vi "AjustTime.vi"(8 "error in (no error)":errorcluster, 10 "Pomiar in":refnum<k34>, 11 "Test in":refnum<k34>) -> (0 "error out":errorcluster, 2 "Pomiar Out":refnum<k34>, 3 "Test Out":refnum<k34>, 4 "First Pomiar":i64, 5 "FirstTest":i64, 7 "End":i64)   [LabVIEW 2019]
uses:
  App/Global_Freq.vi
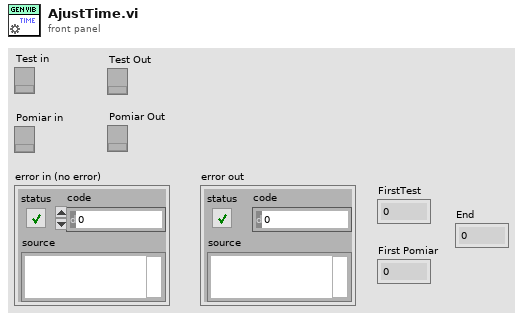
[diagram p1: front panel]
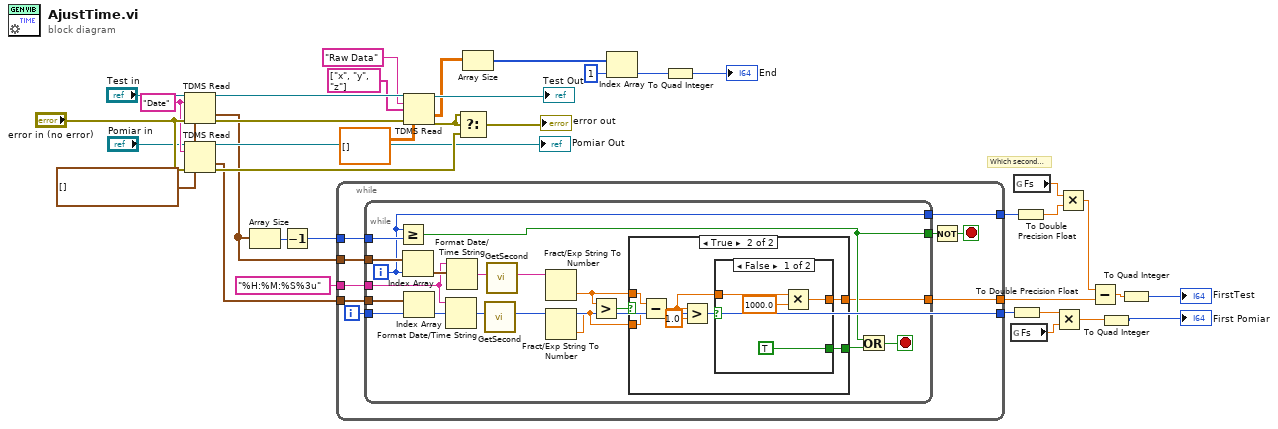
[diagram p0: block diagram]
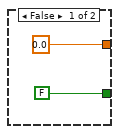
[diagram p2: hidden frame]
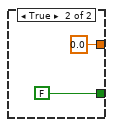
[diagram p3: hidden frame]
diagram:
  w30 = timestamp[] [] ("appended array")
  w34 = "Date" ("group name in")
  # "Which second Test"
  n1 = TDMS Read(0:"Test in", 5:w34, 11:"error in (no error)", 12:w30) -> (4:w29:refnum<k34>, 10:w17:timestamp[], 15:w28:errorcluster)  [unwired: 4 in, 3 out]
  n2 = TDMS Read(0:"Pomiar in", 5:w34, 11:"error in (no error)", 12:w30) -> (4:→"Pomiar Out":refnum<k34>, 10:w19:timestamp[], 15:w35:errorcluster)  [unwired: 4 in, 3 out]
  n3 = Array Size(array=w17) -> (size(s)=w18:i32)
  n4 = Decrement(x=w18) -> (x-1=w16:i32)
  n5 = while {
    tunnel: w19 -> [w46]
    tunnel: w17 -> [w45]
    tunnel: w16 -> [w44]
    tunnel: [w41] -> w15
    tunnel: [w40] -> w12
    tunnel: [w39] -> w8
    tunnel: "%H:%M:%S%3u" ("time format string (%c)") -> [w38]
    i -> [w40]
    stop <- w42 stop-if-true
    n6 = while {
      tunnel: w45 -> [w60]
      tunnel: w46 -> [w59]
      tunnel: w44 -> [w58]
      tunnel: [w55] -> w43
      tunnel: w40 -> [w54]
      tunnel: [w53] -> w41
      tunnel: [w52] -> w39
      tunnel: w38 -> [w47]
      i -> [w53]
      stop <- w56 stop-if-true
      n7 = Greater Or Equal?(x=w53, y=w58) -> (x >= y?=w55:bool)
      n8 = Index Array(array=w60, index=w53) -> (element=w62:timestamp)
      n9 = Index Array(array=w59, index=w54) -> (element=w61:timestamp)
      n10 = Format Date/Time String(time format string (%c)=w47, seconds (now)=w61) -> (date/time string=w49:string)  [unwired: 1 in]
      n11 = Format Date/Time String(time format string (%c)=w47, seconds (now)=w62) -> (date/time string=w51:string)  [unwired: 1 in]
      n12 = call "GetSecond.vi"("String in"=w49) -> ("String out"=w48:string)  [unwired: 10 in]
      n13 = call "GetSecond.vi"("String in"=w51) -> ("String out"=w50:string)  [unwired: 10 in]
      n14 = Fract/Exp String To Number(string=w50) -> (number=w65:dbl)  [unwired: 3 in, 1 out]
      n15 = Fract/Exp String To Number(string=w48) -> (number=w64:dbl)  [unwired: 3 in, 1 out]
      n16 = Greater?(x=w65, y=w64) -> (0:w63:bool)
      n17 = case shown="True" w63 {
        tunnel: w65 -> [_ w71]
        tunnel: w64 -> [_ w70]
        tunnel: [FALSE w69] -> w57
        tunnel: [0.0 w68] -> w52
        frame False {
        }
        frame True {
          n18 = Subtract(x=w71, y=w70) -> (x-y=w72:dbl)
          n19 = Greater?(x=w72, y=1.0) -> (0:w73:bool)
          n20 = case shown="False" w73 {
            tunnel: [TRUE FALSE] -> w69
            tunnel: w72 -> [w77 _]
            tunnel: [w75 0.0] -> w68
            frame False {
              n21 = Multiply(x=w77, y=1000.0) -> (x*y=w75:dbl)
            }
            frame True {
            }
          }
        }
      }
      n22 = Or(x=w55, y=w57) -> (x .or. y?=w56:bool)
    }
    n23 = Not(x=w43) -> (.not. x?=w42:bool)
  }
  n24 = TDMS Read(0:w29, 5:"Raw Data" ("group name in (Untitled)"), 7:string[] ["x", "y", "z"] ("channel name(s) in (Untitled)"), 11:w28, 12:dbl[][] [] ("element")) -> (4:→"Test Out":refnum<k34>, 10:w22:dbl[][], 15:w26:errorcluster)  [unwired: 3 in, 3 out]
  n25 = Select(t=w26, s=w26, f=w35) -> (s? t:f=→"error out":errorcluster)
  n26 = Array Size(array=w22) -> (size(s)=w21:i32[])
  n27 = Index Array(array=w21, index=1) -> (element=w2:i32)
  n28 = To Quad Integer(1:w2) -> (0:→"End":i64)
  n29 = global read "Global_Freq.vi" "Fs"() -> (w10:dbl)
  n30 = To Double Precision Float(number=w12) -> (double precision float=w11:dbl)
  n31 = global read "Global_Freq.vi" "Fs"() -> (w14:dbl)
  n32 = To Double Precision Float(number=w15) -> (double precision float=w13:dbl)
  n33 = Multiply(x=w11, y=w10) -> (x*y=w4:dbl)
  n34 = Multiply(x=w14, y=w13) -> (x*y=w9:dbl)
  n35 = Subtract(x=w9, y=w8) -> (x-y=w6:dbl)
  n36 = To Quad Integer(1:w4) -> (0:→"First Pomiar":i64)
  n37 = To Quad Integer(1:w6) -> (0:→"FirstTest":i64)
